vi "S8300E_memory_databus_WIH.vi"() -> ()   [LabVIEW 2011]
panel:
  out "temp-log":string
  out "Log":string
  out "MSG List":string[](array[string])
  out "VISA resource name out":refnum<visa-resource-name>
  out "Cmd Line":cluster{string, string, "BIST Version":string}[](array[cluster])
  out "BEGIN TIME":u32
  out "進行狀況":string
  # "Error Code:MEM-DATA\nError Code:UART"
  # "2015-6-1"
  # "Memory Data Bus Test (接UART COM9)"
  # "Baud-Rate:115200"
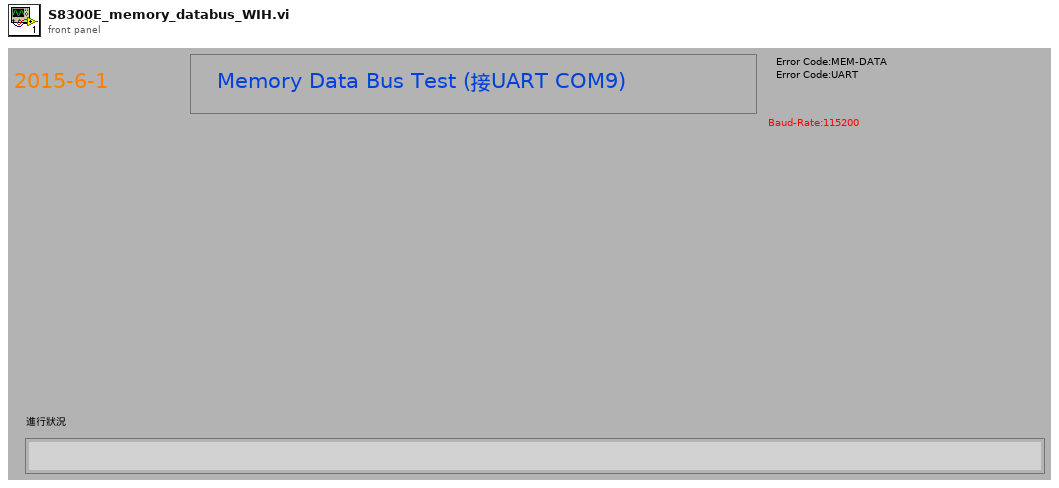
[diagram p1: front panel]
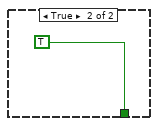
[diagram p4: hidden frame]
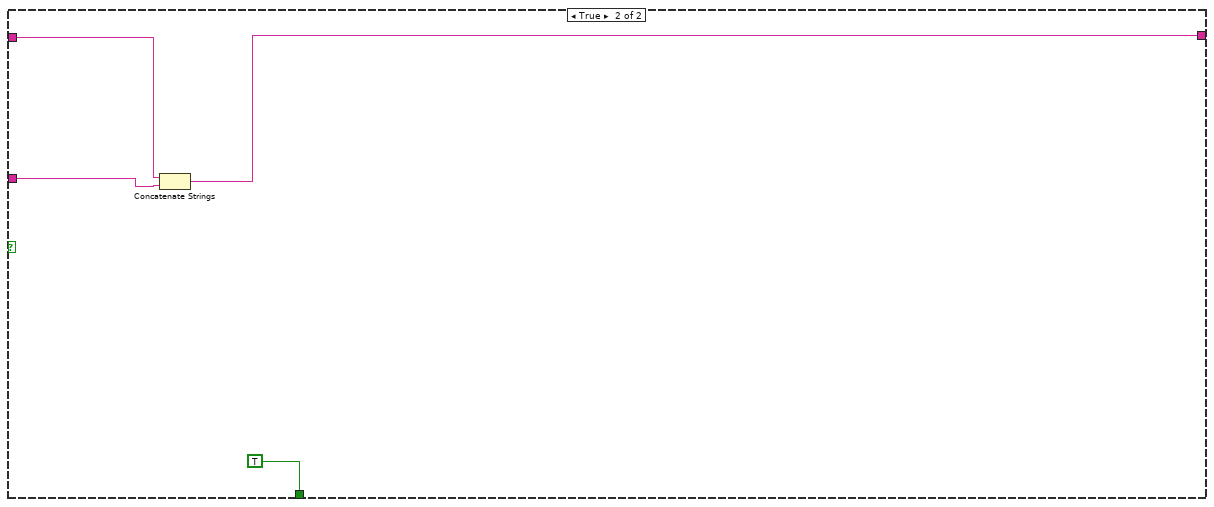
[diagram p6: hidden frame]
diagram:
  n1 = flat-sequence {
    frame #0 {
      n2 = Tick Count (ms)() -> (millisecond timer value=→"BEGIN TIME":u32)
    }
    frame #1 {
      n3 = property on="進行狀況" class="Str"("Blinking"=TRUE) -> ()  [unwired: 2 in, 2 out]
      "進行狀況" <- "進入測試準備中...." ("進行狀況")
    }
    frame #2 {
      n4 = call "SUB_SearchFile_inFolder.vi"("Search Filename in Folder"="S8300E_sfcs_misc.txt") -> ("File Existing True/Flase"=w4:bool)  [unwired: 1 in]
      n5 = case shown="False" w4 {
        frame False {
          n6 = flat-sequence {
            frame #0 {
              n7 = call "Display Message to User"() -> ()  [unwired: 10 in, 2 out]
            }
            frame #1 {
              n8 = call "SUB_Writelog.vi"("Pass/Fail"="Fail:S8300E_memory_databus") -> ()  [unwired: 2 in]
            }
            frame #2 {
              n9 = Quit LabVIEW(quit? (T)=TRUE) -> ()
            }
          }
        }
        frame True {
        }
      }
    }
    frame #3 {
      n10 = Bundle("./mem.sh -d", "PASSED=", "") -> (w10:cluster{string, string, string})  [unwired: 1 in]
      n11 = Build Array(w10) -> (→"Cmd Line":cluster{string, string, string}[])
      n12 = Build Array("正在處理Memory Data Bus 花5秒...") -> (→"MSG List":string[])
    }
    frame #4 {
      n13 = call "SUB_COM1_CLOSE.vi"("VISA resource name"=refnum<visa-resource-name> "COM9") -> ()  [unwired: 3 in]
    }
    frame #5 {
      n14 = call "SUB_COM9_INIT.vi"("baud rate"=u32 115200) -> ("VISA resource name out"=w19:refnum<visa-resource-name>)  [unwired: 1 in, 1 out]
      "VISA resource name out" <- w19
      n15 = call "SUB_COM1Wrt.vi"("VISA resource name"=w19, "write buffer"="\r") -> ("duplicate VISA resource name"=w16:refnum<visa-resource-name>)  [unwired: 1 in, 1 out]
      n16 = call "SUB_ContinueCom1Read.vi"("Numeric"=1200, "duplicate VISA resource name 2"=w16) -> ()  [unwired: 1 in, 3 out]
    }
    frame #6 {
      n17 = while {
        stop <- w32 stop-if-true
        w25 = "\r"
        n18 = local read "VISA resource name out"() -> (w22:refnum<visa-resource-name>)
        n19 = Tick Count (ms)() -> (millisecond timer value=w26:u32)
        n20 = Concatenate Strings(w25, w25, w25, w25) -> (w24:string)
        n21 = call "SUB_ContinueCom1Read.vi"("Numeric"=1200, "duplicate VISA resource name 2"=w22) -> ("duplicate VISA resource name"=w21:refnum<visa-resource-name>)  [unwired: 1 in, 2 out]
        n22 = call "SUB_COM1Wrt.vi"("VISA resource name"=w21, "write buffer"=w24) -> ("duplicate VISA resource name"=w28:refnum<visa-resource-name>)  [unwired: 1 in, 1 out]
        n23 = call "SUB_READ_COM1_FindString_timeout.vi"("Find this String"="S8300E", "Timeout Seccond"=2.0, "Begin time"=w26, "duplicate VISA resource name 2"=w28) -> ("Output String"=w29:string, "Found String"=w30:bool)  [unwired: 1 in, 1 out]
        n24 = case shown="False" w30 {
          tunnel: w29 -> [w37 _]
          tunnel: [w33 TRUE] -> w32
          frame False {
            n25 = call "SUB_YESNO.vi"("Debug View"=w37, "Status"="UART無正確反應!需有S8300E字串") -> ("yes/no"=w36:enum32{"No Selection", "Yes", "No", "None"})  [unwired: 1 in]
            n26 = Equal?(x=w36, y=enum32{"No Selection", "Yes", "No", "None"}."No") -> (x = y?=w34:bool)
            n27 = case shown="True" w34 {
              tunnel: [_ w39] -> w33
              frame False {
              }
              frame True {
                n28 = flat-sequence {
                  tunnel: [w43] -> w39
                  frame #0 {
                    n29 = call "SUB_Writelog.vi"("Pass/Fail"="Fail:S8300E_memory_databus") -> ()  [unwired: 2 in]
                  }
                  frame #1 {
                    n30 = call "SUB_SFCS_SendResult.vi"("ErrorCode"="UART", "PASS_Fail (1/0)"=i8 0) -> ()  [unwired: 1 out]
                  }
                  frame #2 {
                    w43 = TRUE ("quit? (T)")
                    n31 = Quit LabVIEW(quit? (T)=w43) -> ()
                  }
                }
              }
            }
          }
          frame True {
          }
        }
      }
    }
    frame #7 {
      n32 = local read "Cmd Line"() -> (w48:cluster{string, string, "BIST Version":string}[])
      n33 = Array Size(array=w48) -> (size(s)=w47:i32)
      n34 = for {
        N: w47 -> [_]
        shift-right: [w50] -> w45
        shift-left: "" -> [w49]
        i -> [w51]
        n35 = while {
          tunnel: w51 -> [w71]
          tunnel: [w68] -> w50
          tunnel: w49 -> [w67]
          stop <- w66 stop-if-true
          n36 = local read "VISA resource name out"() -> (w55:refnum<visa-resource-name>)
          n37 = local read "Cmd Line"() -> (w70:cluster{string, string, "BIST Version":string}[])
          n38 = call "SUB_ContinueCom1Read.vi"("Numeric"=1200, "duplicate VISA resource name 2"=w55) -> ("duplicate VISA resource name"=w54:refnum<visa-resource-name>)  [unwired: 1 in, 2 out]
          n39 = Index Array(array=w70, index=w71) -> (element=w69:cluster{string, string, "BIST Version":string})
          n40 = Unbundle(w69) -> (w65:string, w58:string)  [unwired: 1 out]
          n41 = Concatenate Strings(w65, "\r") -> (w63:string)
          n42 = call "SUB_COM1Wrt.vi"("VISA resource name"=w54, "write buffer"=w63) -> ("duplicate VISA resource name"=w61:refnum<visa-resource-name>)  [unwired: 1 in, 1 out]
          n43 = Tick Count (ms)() -> (millisecond timer value=w59:u32)
          n44 = call "SUB_READ_COM1_FindString_timeout.vi"("Find this String"=w58, "Timeout Seccond"=10.0, "Begin time"=w59, "duplicate VISA resource name 2"=w61) -> ("Output String"=w62:string)  [unwired: 1 in, 2 out]
          n45 = call "SUB_FindSpecificString.vi"("Find this String"=w58, "String data"=w62) -> ("Found"=w57:bool)  [unwired: 2 in, 1 out]
          n46 = case shown="False" w57 {
            tunnel: w62 -> [w74 w96]
            tunnel: [w73 w95] -> w68
            tunnel: w67 -> [_ w94]
            tunnel: [_ TRUE] -> w66
            frame False {
              w77 = "測試失敗" ("string")
              n47 = local read "進行狀況"() -> (w78:string)
              n48 = Concatenate Strings(w77, w77, "\r", w78) -> (w76:string)
              n49 = call "SUB_YESNO.vi"("Debug View"=w74, "Status"=w76) -> ("yes/no"=w82:enum32{"No Selection", "Yes", "No", "None"})  [unwired: 1 in]
              n50 = Concatenate Strings(w76, "\n", w74) -> (w72:string)
              n51 = Equal?(x=w82, y=enum32{"No Selection", "Yes", "No", "None"}."No") -> (x = y?=w80:bool)
              n52 = case shown="True" w80 {
                tunnel: [w83 _] -> w73
                tunnel: w72 -> [w83 w84]
                frame False {
                }
                frame True {
                  n53 = flat-sequence {
                    tunnel: w84 -> [w86]
                    tunnel: [w92] -> _
                    frame #0 {
                      w87 = "\n"
                      n54 = local read "temp-log"() -> (w88:string)
                      n55 = Concatenate Strings("Fail:S8300E_memory_databus" ("Pass/Fail"), w87, w88, w87, w86) -> (w85:string)
                      n56 = call "SUB_Writelog.vi"("Pass/Fail"=w85) -> ()  [unwired: 2 in]
                    }
                    frame #1 {
                      n57 = call "SUB_SFCS_SendResult.vi"("ErrorCode"="MEM-DATA", "PASS_Fail (1/0)"=i8 0) -> ()  [unwired: 1 out]
                    }
                    frame #2 {
                      w92 = TRUE ("quit? (T)")
                      n58 = Quit LabVIEW(quit? (T)=w92) -> ()
                    }
                  }
                }
              }
            }
            frame True {
              n59 = Concatenate Strings(w94, w96) -> (w95:string)
            }
          }
        }
        "temp-log" <- w50
        n60 = local read "MSG List"() -> (w53:string[])
        n61 = Index Array(array=w53, index=w51) -> (element=w52:string)
        n62 = local write "進行狀況"(w52) -> ()
      }
      "Log" <- w45
    }
    frame #8 {
    }
    frame #9 {
      n63 = call "SUB_COM1_CLOSE.vi"("VISA resource name"=refnum<visa-resource-name> "COM9") -> ()  [unwired: 3 in]
    }
    frame #10 {
      w100 = "***Not Good ***" ("replace string (\"\")")
      n64 = local read "BEGIN TIME"() -> (w109:u32)
      n65 = Tick Count (ms)() -> (millisecond timer value=w108:u32)
      n66 = call "SUB_CAL_TESTTIME.vi"("Test Item name"="S8300E_memory_databus", "Stop tick time"=w108, "Start tick time"=w109) -> ("Test Time output"=w104:string)  [unwired: 2 in]
      n67 = local read "Log"() -> (w105:string)
      n68 = Concatenate Strings("Pass:S8300E_memory_databus", "\n", w105, w104) -> (w99:string)
      n69 = call "SUB_SEARCH_REPLACE_STR.vi"("replace string (\"\")"=w100, "search string"="FAILED", "input string"=w99) -> ("result string"=w102:string)  [unwired: 2 in]
      n70 = call "SUB_SEARCH_REPLACE_STR.vi"("replace string (\"\")"=w100, "search string"="FAIL", "input string"=w102) -> ("result string"=w98:string)  [unwired: 2 in]
      n71 = call "SUB_Writelog.vi"("Pass/Fail"=w98) -> ()  [unwired: 2 in]
    }
    frame #11 {
      n72 = Request Deallocation(TRUE ("flag")) -> ()
    }
    frame #12 {
      n73 = Quit LabVIEW(quit? (T)=TRUE ("stop? (T)")) -> ()
    }
  }
